vi "configure.vi"(8 "error in (no error)":errorcluster, 11 "GenericPlugin in":refnum<class "FPGAWrapperDL090211Galvo.lvclass">) -> (0 "error out":errorcluster, 3 "GenericPlugin out":refnum<class "FPGAWrapperDL090211Galvo.lvclass">)   [LabVIEW 2010, in "FPGAWrapperDL090211Galvo.lvclass"]
doc: "The dynamic dispatch version of this VI loads and displays the configuration file associated with the plug-in object. The user modify and save the configuration data."
uses:
  FPGAWrapperDL090211Galvo.lvclass
  bit_file_enum.ctl
  common_typedefs/pixel_to_host_enum.ctl
  FPGAWrapperDL090211Galvo.lvclass/FPGAWrapperDL090211Galvo.ctl
  common/classes/GenericComponent/GenericComponent/GenericComponent.lvclass
panel:
  in  "pixel-to-host mode":T1
  in  "bit file":T2
  in  "ADC clock phase delay":i32=1 min=1 max=2
  out "configuration":string
  in  "cancelButton":bool
  in  "okButton":bool
  in  "HIFO ADC version":i32=1 min=1 max=2
  # "Configure FPGAWrapperDL090211Galvo"
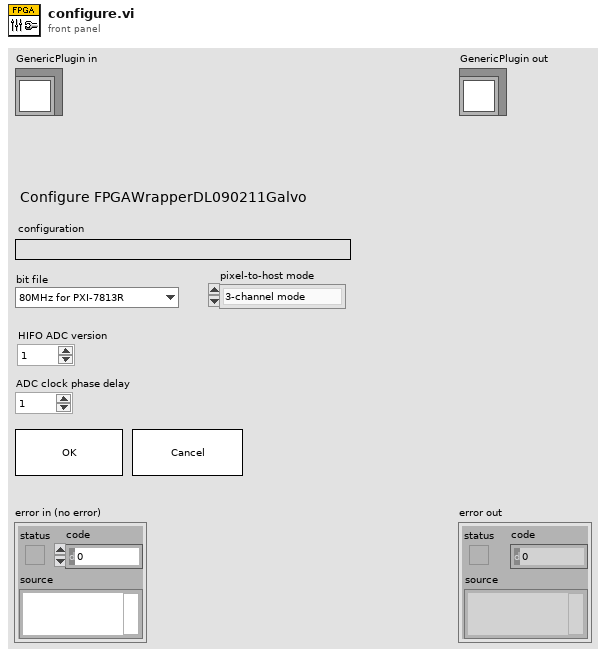
[diagram p1: front panel]
types:
  T1 = typedef "pixel_to_host_enum.ctl" = enum16{"3-channel mode", "4-channel mode"}
  T2 = typedef "FPGAWrapperDL090211Galvo.lvclass/bit_file_enum.ctl" = enum16{"80MHz for PXI-7813R", "120MHz for PXI-7813R"}
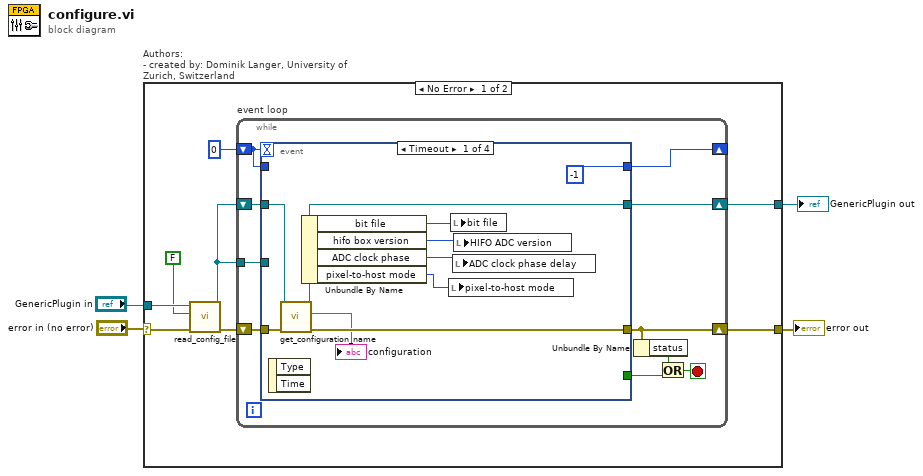
[diagram p0: block diagram]
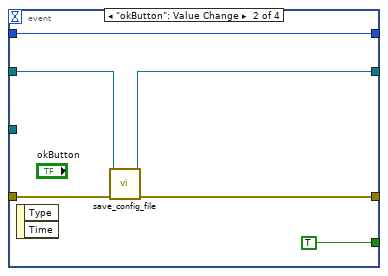
[diagram p2: hidden frame]
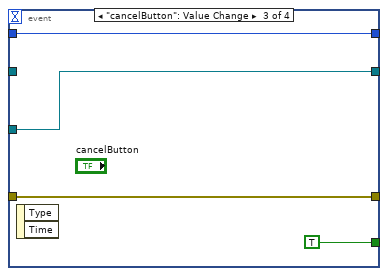
[diagram p3: hidden frame]
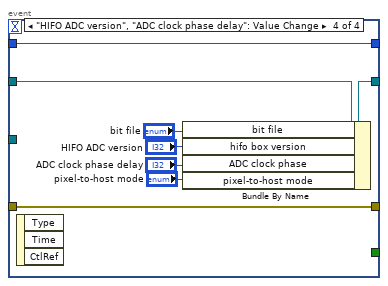
[diagram p4: hidden frame]
diagram:
  n1 = case "Authors: \n- created by: Dominik Langer, University of Zurich, Switzerland" shown="No Error" "error in (no error)" {
    selector: "error in (no error)" -> [w12 w51]
    tunnel: "GenericPlugin in" -> [w10 w52]
    tunnel: [w7 w51] -> w2
    tunnel: [w6 w52] -> w1
    frame No Error {
      n2 = call-dynamic "read_config_file.vi"("error in (no error)"=w12, "force load?"=FALSE, "GenericPlugin in"=w10) -> ("error out"=w11:errorcluster, "GenericPlugin out"=w8:refnum<class "FPGAWrapperDL090211Galvo.lvclass">)  [unwired: 7 in]
      n3 = while "event loop" {
        shift-right: [w18] -> w7
        shift-left: w11 -> [w21]
        shift-right: [w20] -> w6
        shift-left: w8 -> [w22]
        tunnel: w8 -> [w19]
        shift-right: [w13] -> _
        shift-left: 0 -> [w14]
        stop <- w15 stop-if-true
        n4 = event shown="[0] Timeout" {
          selector: _ -> [_ _ _ _]
          dyn-events: _ -> [_ _ _ _]
          timeout: w14 -> [_ _ _ _]
          tunnel: w22 -> [w29 w36 _ w49]
          tunnel: w21 -> [w31 w38 w42 w50]
          tunnel: [w30 w37 w42 w50] -> w18
          tunnel: [w28 w35 w41 w48] -> w20
          tunnel: w19 -> [_ _ w41 _]
          tunnel: [_ TRUE TRUE _] -> w16
          tunnel: w14 -> [_ w33 w39 w45]
          tunnel: [-1 w33 w39 w45] -> w13
          event Timeout {
            n5 = event-data() -> ()  [unwired: 1 in, 2 out]
            n6 = call "get_configuration_name.vi"("error in (no error)"=w31, "GenericPlugin.lvclass in"=w29) -> ("error out"=w30:errorcluster, "configuration name"=→"configuration":string, "GenericPlugin.lvclass out"=w28:refnum<class "FPGAWrapperDL090211Galvo.lvclass">)  [unwired: 7 in]
            n7 = Unbundle By Name(w28) -> ("bit file"=w24:T2, "hifo box version"=w32:i32, "ADC clock phase"=w26:i32, "pixel-to-host mode"=w23:T1)
            n8 = local write "pixel-to-host mode"(w23) -> ()
            n9 = local write "bit file"(w24) -> ()
            n10 = local write "ADC clock phase delay"(w26) -> ()
            n11 = local write "HIFO ADC version"(w32) -> ()
          }
          event "okButton": Value Change {
            n12 = event-data() -> ()  [unwired: 1 in, 2 out]
            n13 = call-dynamic "save_config_file.vi"("error in (no error)"=w38, "GenericPlugin in"=w36) -> ("error out"=w37:errorcluster, "GenericPlugin out"=w35:refnum<class "FPGAWrapperDL090211Galvo.lvclass">)  [unwired: 8 in]
          }
          event "cancelButton": Value Change {
            n14 = event-data() -> ()  [unwired: 1 in, 2 out]
          }
          event "HIFO ADC version", "ADC clock phase delay": Value Change {
            n15 = event-data() -> ()  [unwired: 1 in, 3 out]
            n16 = Bundle By Name(cluster=w49, "bit file"="bit file", "hifo box version"="HIFO ADC version", "ADC clock phase"="ADC clock phase delay", "pixel-to-host mode"="pixel-to-host mode") -> (w48:refnum<class "FPGAWrapperDL090211Galvo.lvclass">)
          }
        }
        n17 = Unbundle By Name(w18) -> ("status"=w17:bool)
        n18 = Or(x=w17, y=w16) -> (x .or. y?=w15:bool)
      }
    }
    frame Error {
    }
  }
  "error out" <- w2
  "GenericPlugin out" <- w1
